vi "Revert User Dialog.vi"(8 "error in (no error)":errorcluster) -> (0 "error out":errorcluster, 2 "Revert":bool)   [LabVIEW 2021, in "TemplateCoreUtilities.lvlib"]
uses:
  TemplateCoreUtilities.lvlib
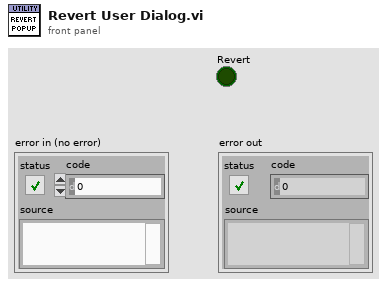
[diagram p1: front panel]
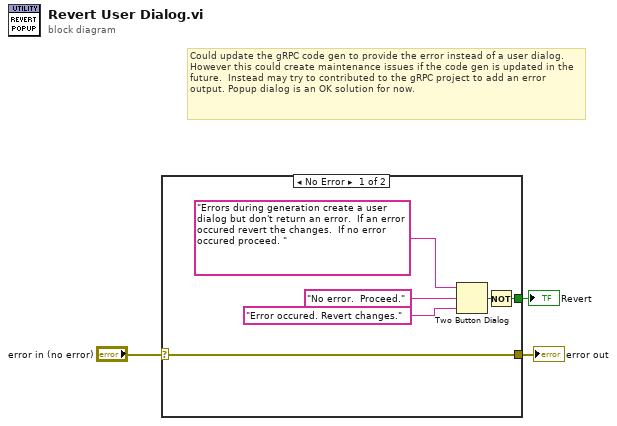
[diagram p0: block diagram]
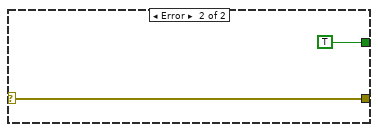
[diagram p2: hidden frame]
diagram:
  # "Could update the gRPC code gen to provide the error instead of a user dialog.  However this could create maintenance issues if the code gen is updated in the future.  Instead may try to contributed to the gRPC project to add an error output. Popup dialog is an OK solution for now."
  n1 = case shown="No Error" "error in (no error)" {
    selector: "error in (no error)" -> [w4 w11]
    tunnel: [w5 TRUE] -> w3
    tunnel: [w4 w11] -> w1
    frame No Error {
      n2 = Two Button Dialog(message="Errors during generation create a user dialog but don't return an error.  If an error occured revert the changes.  If no error occured proceed. ", 1:"Error occured. Revert changes." ("F button name (\"Cancel\")"), 2:"No error.  Proceed." ("T button name (\"OK\")")) -> (T button?=w6:bool)
      n3 = Not(x=w6) -> (.not. x?=w5:bool)
    }
    frame Error {
    }
  }
  "error out" <- w1
  "Revert" <- w3
